vi "get_name.vi"(8 "error in (no error)":errorcluster, 11 "command in":refnum<class "command_generic.lvclass">) -> (0 "error out":errorcluster, 2 "name":string, 3 "command out":refnum<class "command_generic.lvclass">)   [LabVIEW 2015, in "command_generic.lvclass"]
uses:
  command_generic.lvclass
  command_generic.lvclass/command_generic.ctl
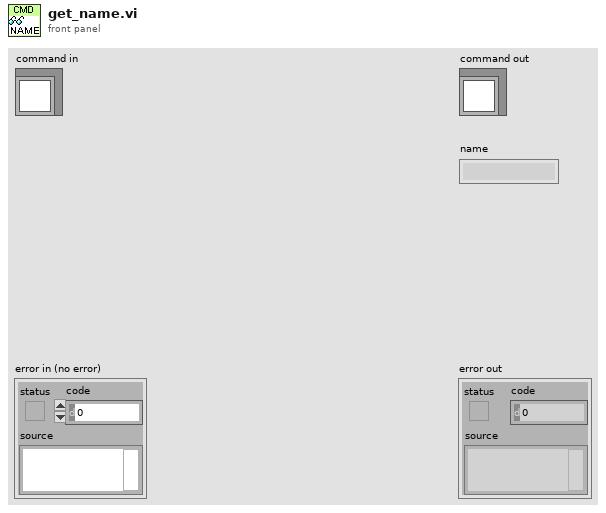
[diagram p1: front panel]
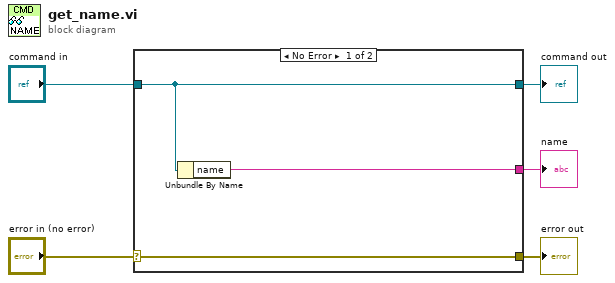
[diagram p0: block diagram]
diagram:
  n1 = case shown="No Error" "error in (no error)" {
    selector: "error in (no error)" -> [w8 w9]
    tunnel: [w8 w9] -> w4
    tunnel: [w7 w10] -> w2
    tunnel: "command in" -> [w7 w10]
    tunnel: [w6 _] -> w1
    frame No Error {
      n2 = Unbundle By Name(w7) -> ("name"=w6:string)
    }
    frame Error {
    }
  }
  "error out" <- w4
  "command out" <- w2
  "name" <- w1
